vi "CFN61G_U8-to-B2-61_v1.vi"(11 "U8_Input":u8[](array[numeric])) -> (3 "Output_Cluster":T1)   [LabVIEW 2017]
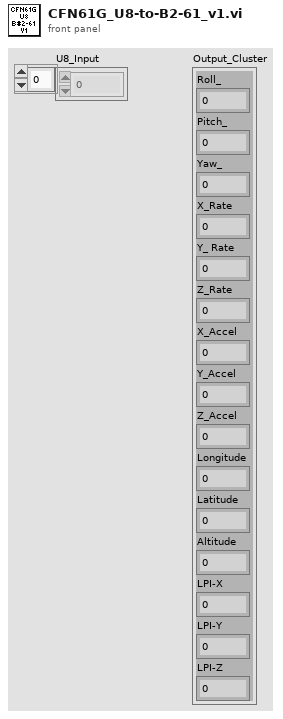
[diagram p1: front panel]
types:
  T1 = cluster{"Roll_":sgl, "Pitch_":sgl, "Yaw_":sgl, "X_Rate":sgl, "Y_ Rate":sgl, "Z_Rate":sgl, "X_Accel":sgl, "Y_Accel":sgl, "Z_Accel":sgl, "Longitude":sgl, "Latitude":sgl, "Altitude":sgl, "LPI-X":sgl, "LPI-Y":sgl, "LPI-Z":sgl}
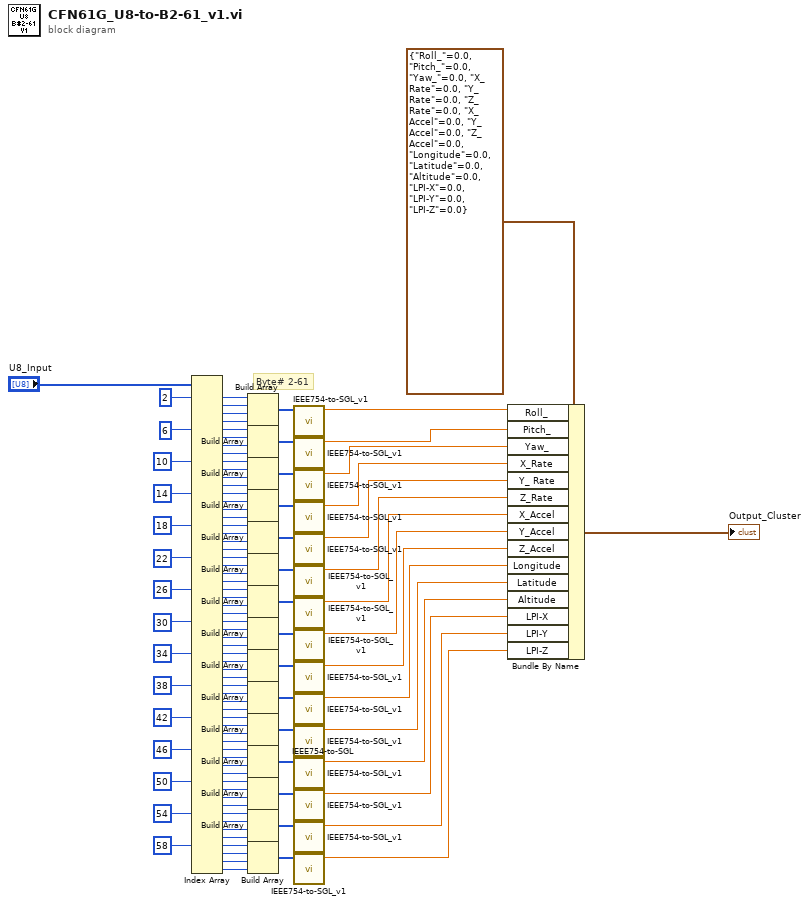
[diagram p0: block diagram]
diagram:
  # "Byte# 2-61"
  n1 = Index Array(array="U8_Input", index #1=2 ("index"), index #5=6 ("index"), index #9=10 ("index"), index #13=14 ("index"), index #17=18 ("index"), index #21=22 ("index"), index #25=26 ("index"), index #29=30 ("index"), index #33=34 ("index"), index #37=38 ("index"), index #41=42 ("index"), index #45=46 ("index"), index #49=50 ("index"), index #53=54 ("index"), index #57=58 ("index")) -> (element #1=w91:u8, element #2=w90:u8, element #3=w89:u8, element #4=w88:u8, element #5=w84:u8, element #6=w83:u8, element #7=w82:u8, element #8=w81:u8, element #9=w80:u8, element #10=w79:u8, element #11=w78:u8, element #12=w77:u8, element #13=w72:u8, element #14=w73:u8, element #15=w71:u8, element #16=w70:u8, element #17=w69:u8, element #18=w68:u8, element #19=w67:u8, element #20=w66:u8, element #21=w65:u8, element #22=w64:u8, element #23=w63:u8, element #24=w62:u8, element #25=w56:u8, element #26=w55:u8, element #27=w54:u8, element #28=w53:u8, element #29=w52:u8, element #30=w51:u8, element #31=w50:u8, element #32=w49:u8, element #33=w48:u8, element #34=w47:u8, element #35=w46:u8, element #36=w45:u8, element #37=w44:u8, element #38=w43:u8, element #39=w42:u8, element #40=w41:u8, element #41=w40:u8, element #42=w39:u8, element #43=w38:u8, element #44=w37:u8, element #45=w36:u8, element #46=w35:u8, element #47=w34:u8, element #48=w33:u8, element #49=w29:u8, element #50=w28:u8, element #51=w27:u8, element #52=w26:u8, element #53=w25:u8, element #54=w24:u8, element #55=w23:u8, element #56=w22:u8, element #57=w21:u8, element #58=w20:u8, element #59=w18:u8, element #60=w19:u8)  [unwired: 45 in]
  n2 = Build Array(w91, w90, w89, w88) -> (w87:u8[])
  n3 = Build Array(w84, w83, w82, w81) -> (w86:u8[])
  n4 = Build Array(w80, w79, w78, w77) -> (w85:u8[])
  n5 = Build Array(w72, w73, w71, w70) -> (w74:u8[])
  n6 = Build Array(w69, w68, w67, w66) -> (w75:u8[])
  n7 = Build Array(w65, w64, w63, w62) -> (w76:u8[])
  n8 = Build Array(w56, w55, w54, w53) -> (w57:u8[])
  n9 = Build Array(w52, w51, w50, w49) -> (w58:u8[])
  n10 = Build Array(w48, w47, w46, w45) -> (w59:u8[])
  n11 = Build Array(w44, w43, w42, w41) -> (w61:u8[])
  n12 = Build Array(w40, w39, w38, w37) -> (w60:u8[])
  n13 = Build Array(w36, w35, w34, w33) -> (w17:u8[])
  n14 = Build Array(w29, w28, w27, w26) -> (w30:u8[])
  n15 = Build Array(w25, w24, w23, w22) -> (w31:u8[])
  n16 = Build Array(w21, w20, w18, w19) -> (w32:u8[])
  n17 = call "IEEE754-to-SGL_v1.vi"("Input_U8"=w87) -> ("Output_SGL"=w94:sgl)  [unwired: 10 in]
  n18 = call "IEEE754-to-SGL_v1.vi"("Input_U8"=w86) -> ("Output_SGL"=w95:sgl)  [unwired: 10 in]
  n19 = call "IEEE754-to-SGL_v1.vi"("Input_U8"=w85) -> ("Output_SGL"=w96:sgl)  [unwired: 10 in]
  n20 = call "IEEE754-to-SGL_v1.vi"("Input_U8"=w74) -> ("Output_SGL"=w97:sgl)  [unwired: 10 in]
  n21 = call "IEEE754-to-SGL_v1.vi"("Input_U8"=w75) -> ("Output_SGL"=w98:sgl)  [unwired: 10 in]
  n22 = call "IEEE754-to-SGL_v1.vi"("Input_U8"=w76) -> ("Output_SGL"=w99:sgl)  [unwired: 10 in]
  n23 = call "IEEE754-to-SGL_v1.vi"("Input_U8"=w57) -> ("Output_SGL"=w100:sgl)  [unwired: 10 in]
  n24 = call "IEEE754-to-SGL_v1.vi"("Input_U8"=w58) -> ("Output_SGL"=w101:sgl)  [unwired: 10 in]
  n25 = call "IEEE754-to-SGL_v1.vi"("Input_U8"=w59) -> ("Output_SGL"=w102:sgl)  [unwired: 10 in]
  n26 = call "IEEE754-to-SGL_v1.vi"("Input_U8"=w61) -> ("Output_SGL"=w103:sgl)  [unwired: 10 in]
  n27 = call "IEEE754-to-SGL_v1.vi"("Input_U8"=w60) -> ("Output_SGL"=w104:sgl)  [unwired: 10 in]
  n28 = call "IEEE754-to-SGL_v1.vi"("Input_U8"=w17) -> ("Output_SGL"=w105:sgl)  [unwired: 10 in]
  n29 = call "IEEE754-to-SGL.vi"() -> ()  [unwired: 11 in, 1 out]
  n30 = call "IEEE754-to-SGL_v1.vi"("Input_U8"=w30) -> ("Output_SGL"=w106:sgl)  [unwired: 10 in]
  n31 = call "IEEE754-to-SGL_v1.vi"("Input_U8"=w31) -> ("Output_SGL"=w107:sgl)  [unwired: 10 in]
  n32 = call "IEEE754-to-SGL_v1.vi"("Input_U8"=w32) -> ("Output_SGL"=w108:sgl)  [unwired: 10 in]
  n33 = Bundle By Name(cluster=T1 {"Roll_"=0.0, "Pitch_"=0.0, "Yaw_"=0.0, "X_Rate"=0.0, "Y_ Rate"=0.0, "Z_Rate"=0.0, "X_Accel"=0.0, "Y_Accel"=0.0, "Z_Accel"=0.0, "Longitude"=0.0, "Latitude"=0.0, "Altitude"=0.0, "LPI-X"=0.0, "LPI-Y"=0.0, "LPI-Z"=0.0}, "Roll_"=w94, "Pitch_"=w95, "Yaw_"=w96, "X_Rate"=w97, "Y_ Rate"=w98, "Z_Rate"=w99, "X_Accel"=w100, "Y_Accel"=w101, "Z_Accel"=w102, "Longitude"=w103, "Latitude"=w104, "Altitude"=w105, "LPI-X"=w106, "LPI-Y"=w107, "LPI-Z"=w108) -> (→"Output_Cluster":T1)
